vi "UtilityLib.string dialog.vi"(0 "title":string, 5 "captions":string[](array[string]), 7 "helpText":string[](array[string]), 9 "initialValue":string[](array[string]), 11 "error in (no error)":errorcluster) -> (4 "cancelled":bool, 6 "strings":string[](array[string]), 8 "nOfStrings":i32, 15 "error out":errorcluster)   [LabVIEW 2014, in "UtilityLib.lvlib"]
doc: "lets the user select a name from a string"
uses:
  UtilityLib.lvlib
panel:
  in  "string10":string
  in  "string9":string
  in  "string8":string
  in  "string7":string
  in  "string6":string
  in  "string5":string
  in  "string4":string caption="sqlServerNode"
  in  "string3":string caption="Data Source (ODBC)"
  in  "string2":string caption="systemID"
  in  "string1":string caption="domainName"
  in  "Cancel":bool
  in  "OK Button":bool
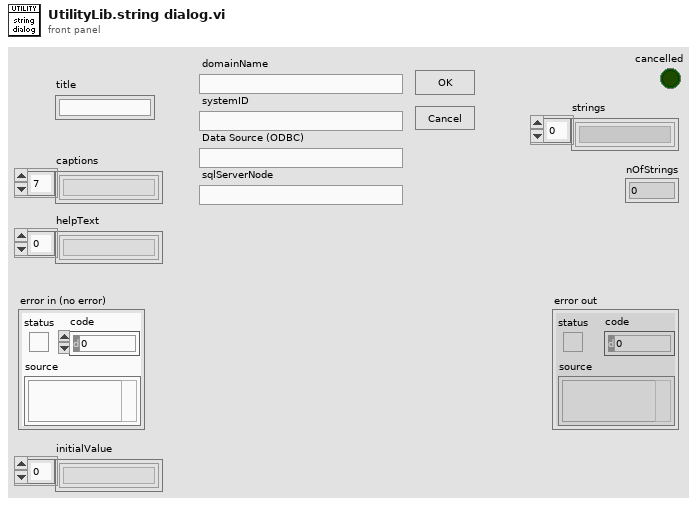
[diagram p1: front panel]
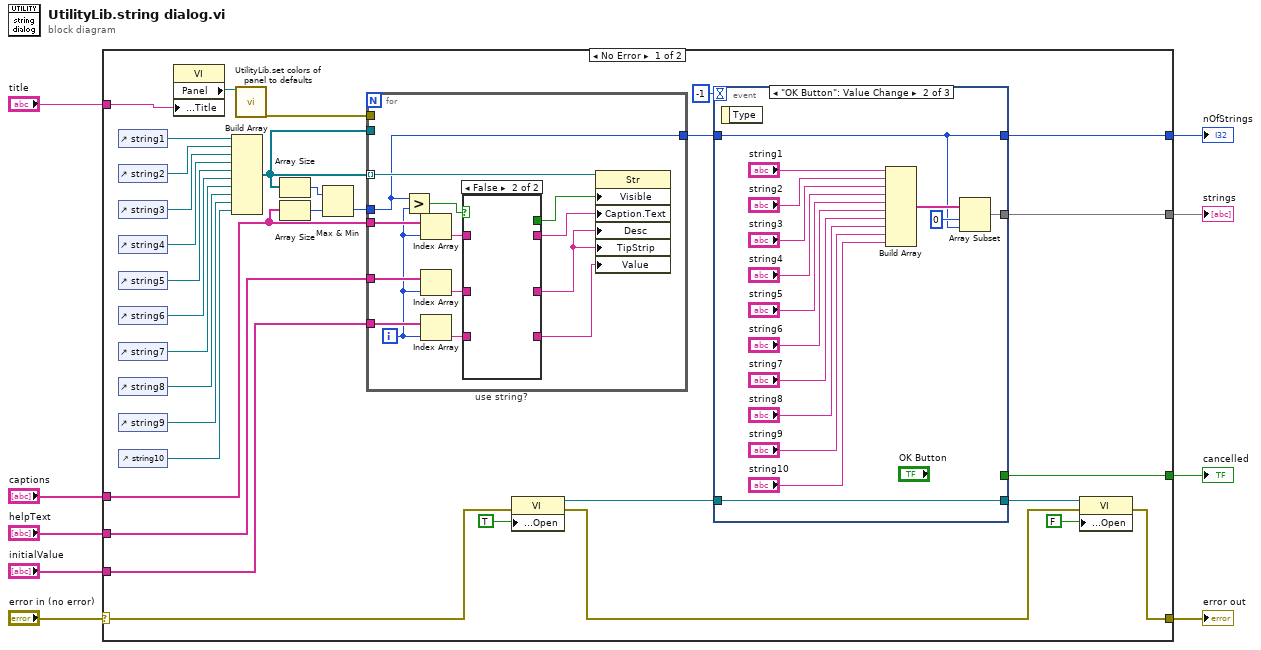
[diagram p0: block diagram]
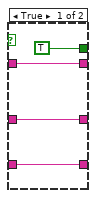
[diagram p2: hidden frame]
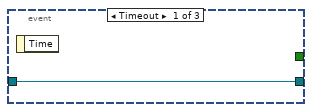
[diagram p3: hidden frame]
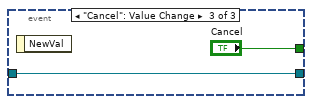
[diagram p4: hidden frame]
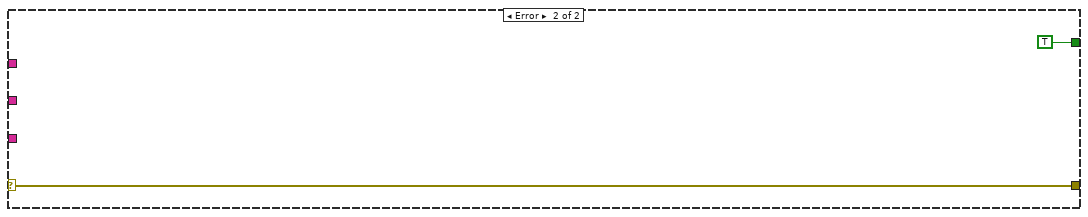
[diagram p5: hidden frame]
diagram:
  n1 = case shown="No Error" "error in (no error)" {
    selector: "error in (no error)" -> [w10 w79]
    tunnel: [w36 TRUE ("Cancel")] -> w9
    tunnel: "helpText" -> [w25 _]
    tunnel: [w24 _] -> w7
    tunnel: [w23 _] -> w6
    tunnel: [w22 w79] -> w5
    tunnel: "title" -> [w18 _]
    tunnel: "initialValue" -> [w17 _]
    tunnel: "captions" -> [w12 _]
    frame No Error {
      n2 = control-ref of="string1"() -> (w35:refnum<vi>)
      n3 = control-ref of="string2"() -> (w34:refnum<vi>)
      n4 = control-ref of="string3"() -> (w33:refnum<vi>)
      n5 = control-ref of="string4"() -> (w32:refnum<vi>)
      n6 = control-ref of="string5"() -> (w31:refnum<vi>)
      n7 = control-ref of="string6"() -> (w30:refnum<vi>)
      n8 = control-ref of="string7"() -> (w29:refnum<vi>)
      n9 = control-ref of="string8"() -> (w28:refnum<vi>)
      n10 = control-ref of="string9"() -> (w27:refnum<vi>)
      n11 = control-ref of="string10"() -> (w26:refnum<vi>)
      n12 = property class="VI"("Front Panel.Title"=w18) -> ("Panel"=w20:refnum<vi>)  [unwired: 2 in, 2 out]
      n13 = Build Array(w35, w34, w33, w32, w31, w30, w29, w28, w27, w26) -> (w13:refnum<vi>[])
      n14 = call "UtilityLib.set colors of panel to defaults.vi"("Front Panel"=w20) -> ("error out"=w19:errorcluster)  [unwired: 18 in]
      n15 = Array Size(array=w13) -> (size(s)=w15:i32)
      n16 = Array Size(array=w12) -> (size(s)=w14:i32)
      n17 = Max & Min(x=w15, y=w14) -> (min(x,y)=w11:i32)  [unwired: 1 out]
      n18 = for {
        tunnel: w13 -> [w55] mode=indexing
        tunnel: w12 -> [w46]
        tunnel: w25 -> [w52]
        tunnel: w19 -> [_]
        tunnel: w17 -> [w47]
        tunnel: w13 -> [_]
        tunnel: [w44] -> w16
        tunnel: w11 -> [w44]
        i -> [w43]
        n19 = Greater?(x=w44, y=w43) -> (0:w45:bool)
        n20 = Index Array(array=w46, index=w43) -> (element=w42:string)
        n21 = Index Array(array=w52, index=w43) -> (element=w51:string)
        n22 = Index Array(array=w47, index=w43) -> (element=w49:string)
        n23 = case "use string?" shown="False" w45 {
          tunnel: [TRUE _] -> w54
          tunnel: [w56 _] -> w53
          tunnel: [w58 _] -> w50
          tunnel: w51 -> [w58 _]
          tunnel: w49 -> [w57 _]
          tunnel: [w57 _] -> w48
          tunnel: w42 -> [w56 _]
          frame True {
          }
          frame False {
          }
        }
        n24 = property class="Str"(reference=w55, "Visible"=w54, "Caption.Text"=w53, "Desc"=w50, "TipStrip"=w50, "Value"=w48) -> ()  [unwired: 1 in, 2 out]
      }
      n25 = property class="VI"(error in=w10, "Front Panel Window:Open"=TRUE) -> (reference out=w40:refnum<vi>, error out=w37:errorcluster)  [unwired: 1 in]
      n26 = event shown="[1] \"OK Button\": Value Change" {
        selector: _ -> [_ _ _]
        dyn-events: _ -> [_ _ _]
        timeout: -1 -> [_ _ _]
        tunnel: [w60 w75 w77] -> w38
        tunnel: w40 -> [w60 w75 w77]
        tunnel: [_ _ "Cancel"] -> w36
        tunnel: w16 -> [_ w62 _]
        tunnel: [_ w62 _] -> w24
        tunnel: [_ w61 _] -> w23
        event Timeout {
          n27 = event-data() -> ()  [unwired: 1 in, 1 out]
        }
        event "OK Button": Value Change {
          n28 = event-data() -> ()  [unwired: 1 in, 1 out]
          n29 = Build Array("string1", "string2", "string3", "string4", "string5", "string6", "string7", "string8", "string9", "string10") -> (w64:string[])
          n30 = Array Subset(array=w64, index=0, length=w62) -> (w61:string[])
        }
        event "Cancel": Value Change {
          n31 = event-data() -> ()  [unwired: 1 in, 1 out]
        }
      }
      n32 = property class="VI"(reference=w38, error in=w37, "Front Panel Window:Open"=FALSE) -> (error out=w22:errorcluster)  [unwired: 1 out]
    }
    frame Error {
    }
  }
  "error out" <- w5
  "cancelled" <- w9
  "strings" <- w6
  "nOfStrings" <- w7
